vi "Get CRI.vi"(8 "error in (no error)":errorcluster, 9 "Hi Res?":bool, 10 "IRRAD Input Parameters":T1, 11 "Color Parameters in":T2) -> (0 "error out":errorcluster, 2 "IRRAD Input Parameters out":T1, 3 "Color Parameters out":T2)   [LabVIEW 2013, in "AvaSpec.lvlib" / "AVSirrad_support.lvlib"]
uses:
  AVSirrad_support.lvlib
  AvaSpec Color Parameters.ctl
  IRRAD input parameters.ctl
  Libraries/IRRAD-DLL/AVSirrad.lvlib
  AvaSpec.lvlib
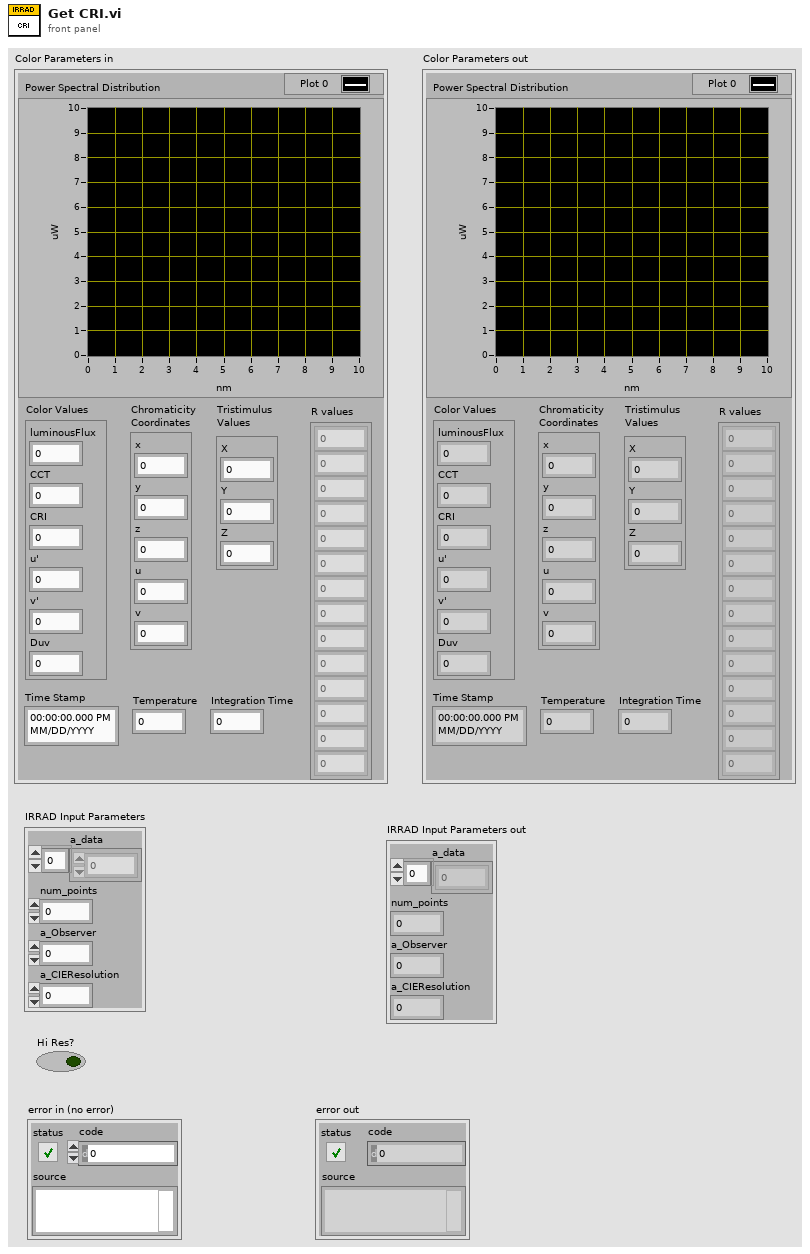
[diagram p1: front panel]
types:
  T1 = typedef "IRRAD input parameters.ctl" = cluster{"a_data":dbl[], "num_points":i32, "a_Observer":u8, "a_CIEResolution":u8}
  T2 = typedef "AvaSpec.lvlib/AvaSpec Color Parameters.ctl" = cluster{"Power Spectral Distribution":cluster{"X":dbl, "Y":dbl}[], "Color Values":cluster{"luminousFlux":dbl, "CCT":dbl, "CRI":dbl, "u'":dbl, "v'":dbl, "Duv":dbl}, "R values":dbl[], "Chromaticity \nCoordinates":cluster{"x":dbl, "y":dbl, "z":dbl, "u":dbl, "v":dbl}, "Tristimulus \nValues":cluster{"X":dbl, "Y":dbl, "Z":dbl}, "Time Stamp":timestamp, "Temperature":dbl, "Integration Time":dbl}
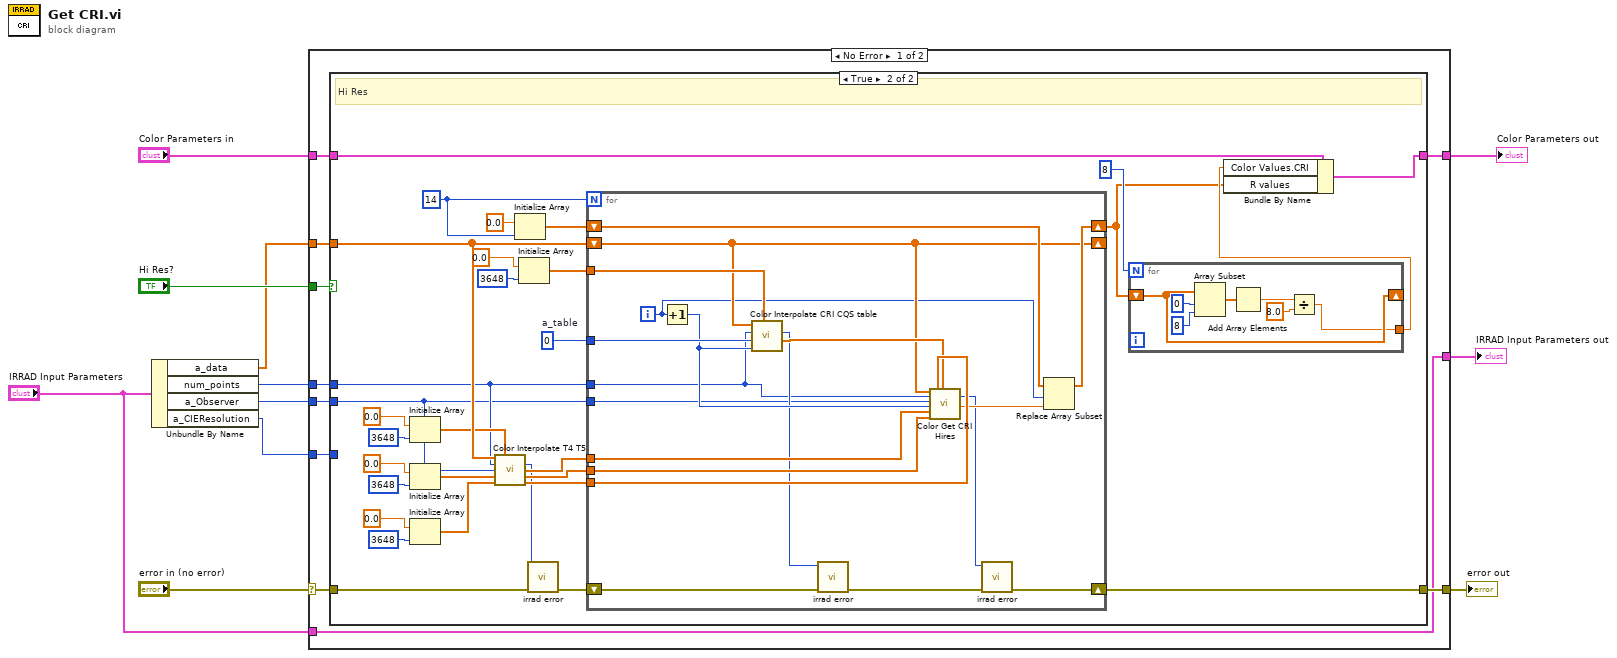
[diagram p0: block diagram]
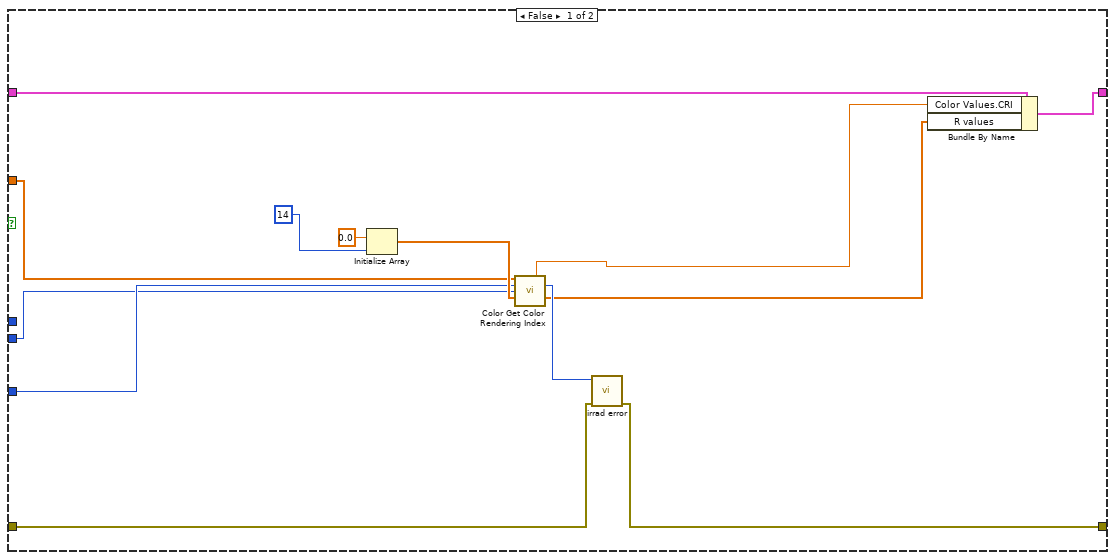
[diagram p2: hidden frame]
diagram:
  n1 = Unbundle By Name("IRRAD Input Parameters") -> ("a_data"=w6:dbl[], "num_points"=w5:i32, "a_Observer"=w4:u8, "a_CIEResolution"=w3:u8)
  n2 = case shown="No Error" "error in (no error)" {
    selector: "error in (no error)" -> [w18 w94]
    tunnel: w6 -> [w21 _]
    tunnel: "Hi Res?" -> [w20 _]
    tunnel: [w19 w94] -> w10
    tunnel: "Color Parameters in" -> [w17 w93]
    tunnel: [w16 w93] -> w7
    tunnel: w5 -> [w15 _]
    tunnel: w4 -> [w14 _]
    tunnel: w3 -> [w13 _]
    tunnel: [w12 w92] -> w2
    tunnel: "IRRAD Input Parameters" -> [w12 w92]
    frame No Error {
      n3 = case shown="True" w20 {
        tunnel: w21 -> [w31 w65]
        tunnel: w18 -> [w30 w42]
        tunnel: [w29 w44] -> w19
        tunnel: w17 -> [w27 w40]
        tunnel: [w26 w39] -> w16
        tunnel: w15 -> [_ w36]
        tunnel: w14 -> [w22 w35]
        tunnel: w13 -> [w23 _]
        frame False {
          n4 = Initialize Array(0.0 ("element"), 14 ("dimension size")) -> (w32:dbl[])
          n5 = call "Color Get Color Rendering Index.vi"("a_data"=w31, "a_CIEResolution"=w23, "a_Observer"=w22, "R_Values"=w32) -> ("CRI out"=w24:dbl, "function return"=w28:i16, "R_Values out"=w25:dbl[])  [unwired: 7 in, 2 out]
          n6 = call "irrad error.vi"("error in (no error)"=w30, "Output Value"=w28) -> ("error out"=w29:errorcluster)  [unwired: 9 in]
          n7 = Bundle By Name(cluster=w27, "Color Values.CRI"=w24, "R values"=w25) -> (w26:T2)
        }
        frame True {
          w59 = u8 0  # a_table
          w58 = 14 ("dimension size")
          # "Hi Res"
          n8 = Initialize Array(0.0 ("element"), 3648 ("dimension size")) -> (w54:dbl[])
          n9 = Initialize Array(0.0 ("element"), 3648 ("dimension size")) -> (w52:dbl[])
          n10 = Initialize Array(0.0 ("element"), 3648 ("dimension size")) -> (w53:dbl[])
          n11 = call "Color Interpolate T4 T5.vi"("a_data"=w65, "a_zarray"=w54, "a_NumPoints"=w36, "a_Observer"=w35, "a_xarray"=w52, "a_yarray"=w53) -> ("function return"=w43:i16, "a_xarray out"=w55:dbl[], "a_yarray out"=w56:dbl[], "a_zarray out"=w57:dbl[])  [unwired: 4 in, 2 out]
          n12 = Initialize Array(0.0 ("element"), w58) -> (w63:dbl[])
          n13 = Initialize Array(0.0 ("element"), 3648 ("dimension size")) -> (w61:dbl[])
          n14 = call "irrad error.vi"("error in (no error)"=w42, "Output Value"=w43) -> ("error out"=w41:errorcluster)  [unwired: 9 in]
          n15 = for {
            N: w58 -> [_]
            tunnel: w55 -> [w91]
            tunnel: w56 -> [w90]
            tunnel: w57 -> [w89]
            tunnel: w59 -> [w88]
            tunnel: w61 -> [w87]
            shift-right: [w82] -> w37
            shift-left: w63 -> [w84]
            shift-right: [w81] -> _
            shift-left: w65 -> [w81]
            shift-right: [w75] -> w44
            shift-left: w41 -> [w77]
            tunnel: w36 -> [w73]
            tunnel: w35 -> [w74]
            i -> [w80]
            n16 = Increment(x=w80) -> (x+1=w85:i32)
            n17 = call "Color Interpolate CRI CQS table.vi"("a_tabelarray"=w87, "a_CRI_CQSsample"=w85, "a_table"=w88, "a_NumInter"=w73, "a_data"=w81) -> ("a_tabelarray out"=w86:dbl[], "function return"=w78:i16)  [unwired: 1 in, 2 out]
            n18 = call "irrad error.vi"("error in (no error)"=w77, "Output Value"=w78) -> ("error out"=w76:errorcluster)  [unwired: 9 in]
            n19 = call "Color Get CRI Hires.vi"("a_data"=w81, "a_NumPoints"=w73, "a_Observer"=w74, "a_samplenumber"=w85, "a_xarray"=w91, "a_yarray"=w90, "a_zarray"=w89, "a_CRItable"=w86) -> ("a_Rvalue out"=w83:dbl, "function return"=w79:i16)  [unwired: 4 in, 6 out]
            n20 = call "irrad error.vi"("error in (no error)"=w76, "Output Value"=w79) -> ("error out"=w75:errorcluster)  [unwired: 9 in]
            n21 = Replace Array Subset(array=w84, new element=w83, index=w80) -> (w82:dbl[])
          }
          n22 = for {
            N: 8 -> [_]
            shift-right: [w70] -> _
            shift-left: w37 -> [w70]
            tunnel: [w66] -> w38
            n23 = Array Subset(array=w70, index=0, length=8) -> (w69:dbl[])
            n24 = Add Array Elements(numeric array=w69) -> (sum=w72:dbl)
            n25 = Divide(x=w72, y=8.0) -> (x/y=w66:dbl)
          }
          n26 = Bundle By Name(cluster=w40, "Color Values.CRI"=w38, "R values"=w37) -> (w39:T2)
        }
      }
    }
    frame Error {
    }
  }
  "error out" <- w10
  "Color Parameters out" <- w7
  "IRRAD Input Parameters out" <- w2
